vi "Resize.vi"(0 "image in":refnum<class "MSC Image.lvclass">, 1 "Size":T2, 2 "Interpolation Method":T1 items=["Nearest Neighbor"=0, "Linear"=1, "Cubic"=2, "Area"=3, "LANCZOS4"=4, "MAX"=7, "Inverse Map"=16], 5 "error in (no error)":errorcluster) -> (14 "image out":refnum<class "MSC Image.lvclass">, 19 "error out":errorcluster)   [LabVIEW 2016, in "MSC Image.lvclass"]
doc: "Resizes the image to the selected size."
uses:
  MSC Image.lvclass
  Dependencies/x86/MSC I Process32.dll
  controls/Size.ctl
  controls/Resize Interpolation Method.ctl
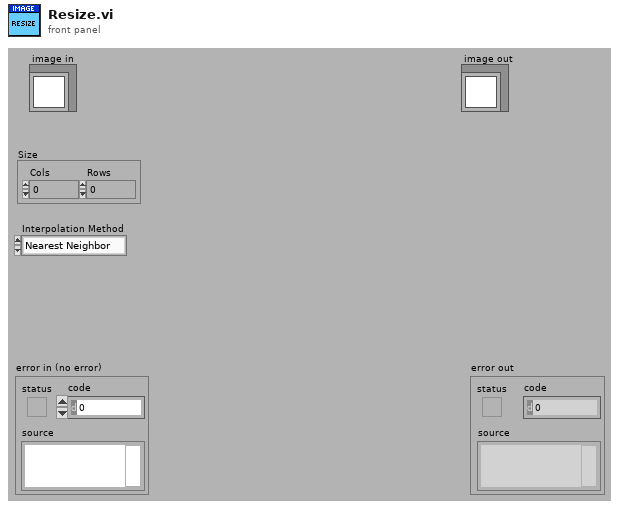
[diagram p1: front panel]
types:
  T1 = typedef "MSC Image.lvclass/Resize Interpolation Method.ctl" = i32
  T2 = typedef "MSC Image.lvclass/Size.ctl" = cluster{"Cols":i32, "Rows":i32}
  T3 = typedef "Image.ctl" = cluster{"Pointer":u64, "Size":T4, "Image Type":T5, "Time Stamp":timestamp, "Variant":variant}
  T4 = typedef "Size.ctl" = cluster{"Cols":i32, "Rows":i32}
  T5 = typedef "Image Type.ctl" = i32
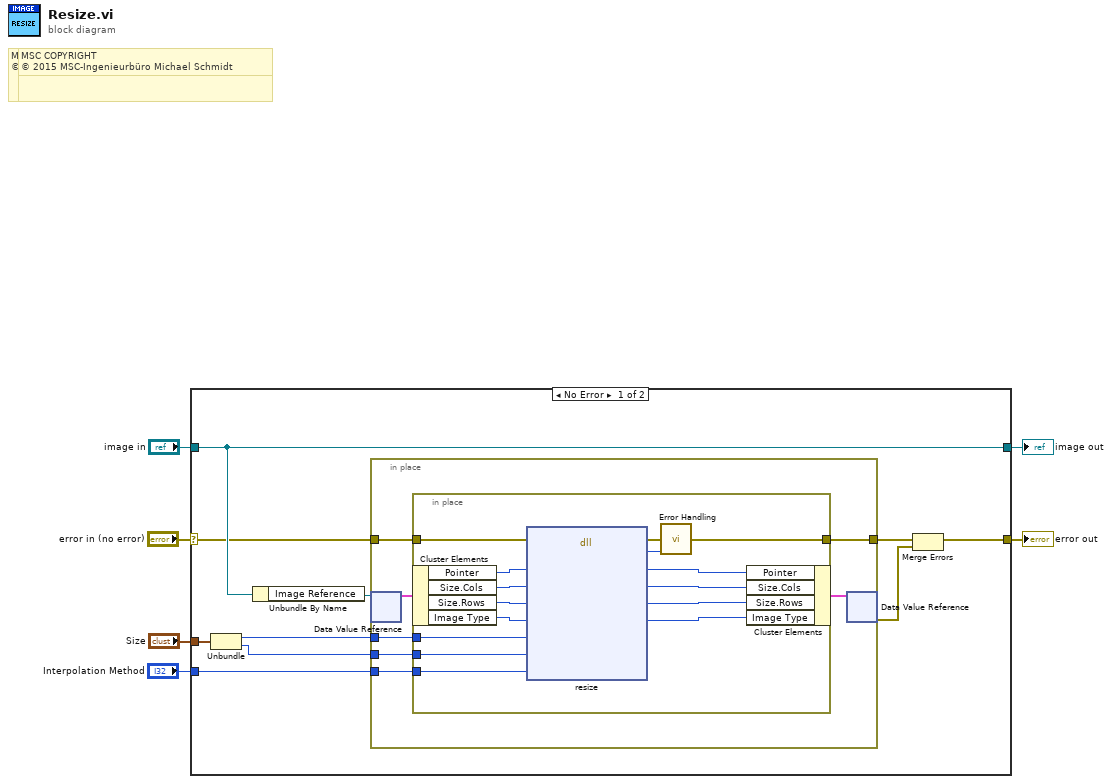
[diagram p0: block diagram]
diagram:
  # "MSC COPYRIGHT\n© 2016 MSC-Ingenieurbüro Michael Schmidt"
  # "MSC COPYRIGHT\n© 2016 MSC-Ingenieurbüro Michael Schmidt"
  # "MSC COPYRIGHT\n© 2015 MSC-Ingenieurbüro Michael Schmidt"
  # "MSC COPYRIGHT\n© 2015 MSC-Ingenieurbüro Michael Schmidt"
  n1 = case shown="No Error" "error in (no error)" {
    selector: "error in (no error)" -> [w12 w40]
    tunnel: [w11 w40] -> w5
    tunnel: [w16 w39] -> w3
    tunnel: "image in" -> [w16 w39]
    tunnel: "Size" -> [w10 _]
    tunnel: "Interpolation Method" -> [w7 _]
    frame No Error {
      n2 = Unbundle(w10) -> ("Cols"=w9:i32, "Rows"=w8:i32)
      n3 = Unbundle By Name(w16) -> ("Image Reference"=w15:refnum<data-value>)
      n4 = in-place {
        in-place-border: w12 -> [w21]
        in-place-border: [w20] -> w14
        in-place-border: w9 -> [w19]
        in-place-border: w8 -> [w18]
        in-place-border: w7 -> [w17]
        n5 = in-place-dvr #1(w15) -> (w22:T3)  [unwired: 1 out]
        n6 = in-place {
          in-place-border: w21 -> [w37]
          in-place-border: [w38] -> w20
          in-place-border: w19 -> [w26]
          in-place-border: w18 -> [w25]
          in-place-border: w17 -> [w24]
          n7 = in-place-cluster #2(w22) -> ("Pointer"=w34:u64, "Size.Cols"=w31:i32, "Size.Rows"=w30:i32, "Image Type"=w28:T5)
          n8 = dll-call lib="C:/Users/MSC/LabVIEW Projekte/LV 2014/MSC I-Process/user.lib/MSC-I Process/Dependencies/x86/MSC I Process*.dll" fn="resize"(error in=w37, "pointer"=w34, "cols"=w31, "rows"=w30, "type"=w28, "colsTo"=w26, "rowsTo"=w25, "interpolationMethod"=w24) -> (error out=w36:errorcluster, "error"=w35:i32, "pointer"=w33:u64, "cols"=w32:i32, "rows"=w29:i32, "type"=w27:i32)  [unwired: 5 in, 1 out]
          n9 = call "Error Handling.vi"("error in (no error)"=w36, "return type"=w35) -> ("error out"=w38:errorcluster)  [unwired: 12 in, 1 out]
          n10 = in-place-cluster #2("Pointer"=w33, "Size.Cols"=w32, "Size.Rows"=w29, "Image Type"=w27) -> (w23:T3)
        }
        n11 = in-place-dvr #1(w23) -> (w13:errorcluster)  [unwired: 1 out]
      }
      n12 = Merge Errors(w14, w13) -> (w11:errorcluster)
    }
    frame Error {
    }
  }
  "error out" <- w5
  "image out" <- w3
